vi "draw_rectangles.vi"(0 "Rectangle Array":dbl[][](array[numeric]), 1 "Robot Properties":T1, 2 "Sim Car.lvclass":refnum<class "Car.lvclass">) -> (7 "Map Picture":picture)   [LabVIEW 2015]
uses:
  Robot.ctl
  class/Car.lvclass
panel:
  out "x*y":dbl[](array[numeric])
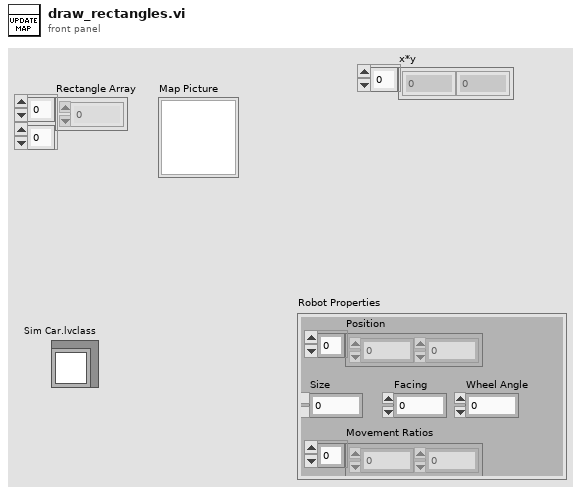
[diagram p1: front panel]
types:
  T1 = typedef "Robot.ctl" = cluster{"Position":dbl[], "Size":dbl, "Facing":dbl, "Movement Ratios":dbl[], "Wheel Angle":dbl}
  T2 = cluster{"Width":i16, "Style":enum32{"Solid", "Dash", "Dot", "DashDot", "DashDotDot"}}
  T3 = cluster{"Rectangle Array[0]":dbl, "Rectangle Array[1]":dbl, "Rectangle Array[2]":dbl, "Rectangle Array[3]":dbl}
  T4 = cluster{"Width":u16, "Style":enum32{"Solid", "Dash", "Dot", "DashDot", "DashDotDot"}}
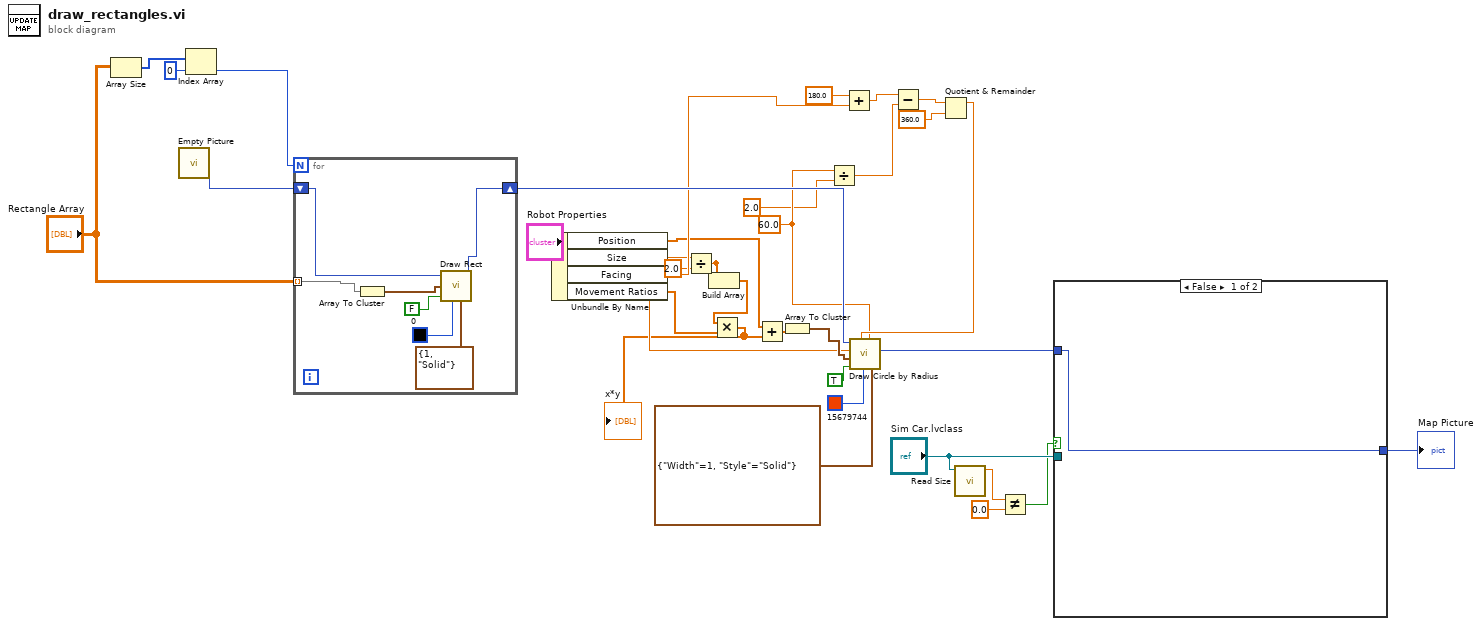
[diagram p0: block diagram]
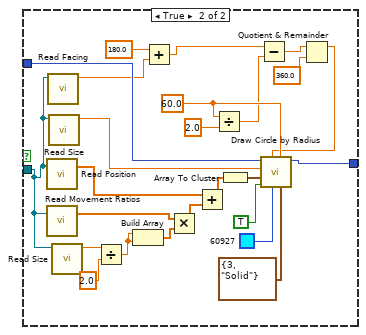
[diagram p2: hidden frame]
diagram:
  w19 = 60.0 ("arc size(360)")
  n1 = Array Size(array="Rectangle Array") -> (size(s)=w31:i32[])
  n2 = call "Empty Picture"() -> ("empty picture"=w34:picture)
  n3 = Index Array(array=w31, index=0) -> (element=w33:i32)
  n4 = for {
    N: w33 -> [_]
    tunnel: "Rectangle Array" -> [w41] mode=indexing
    shift-right: [w35] -> w29
    shift-left: w34 -> [w39]
    n5 = Array To Cluster(array=w41) -> (cluster=w40:T3)
    n6 = call <vilib>:"Draw Rect.vi"("picture"=w39, "rect"=w40, "fill?(F)"=FALSE, "color(black)"=u32 0, "pen"=T2 {"Width"=1, "Style"=enum."Solid"}) -> ("new picture"=w35:picture)  [unwired: 4 in]
  }
  n7 = Unbundle By Name("Robot Properties") -> ("Position"=w13:dbl[], "Size"=w11:dbl, "Facing"=w24:dbl, "Movement Ratios"=w7:dbl[])
  n8 = Divide(x=w11, y=2.0) -> (x/y=w10:dbl)
  n9 = Build Array(w10, w10) -> (w8:dbl[])
  n10 = Multiply(x=w8, y=w7) -> (x*y=w9:dbl[])
  "x*y" <- w9
  n11 = Add(x=w13, y=w9) -> (x+y=w14:dbl[])
  n12 = Array To Cluster(array=w14) -> (cluster=w15:cluster{"[0]":dbl, "[1]":dbl})
  n13 = Divide(x=w19, y=2.0) -> (x/y=w17:dbl)
  n14 = Add(x=180.0, y=w24) -> (x+y=w23:dbl)
  n15 = Subtract(x=w23, y=w17) -> (x-y=w22:dbl)
  n16 = Quotient & Remainder(x=w22, y=360.0) -> (x-y*floor(x/y)=w20:dbl)  [unwired: 1 out]
  n17 = call <vilib>:"Draw Circle by Radius.vi"("pen"=T2 {"Width"=1, "Style"=enum."Solid"}, "arc size(360)"=w19, "color(black)"=u32 15679744, "start angle(0)"=w20, "fill?(F)"=TRUE, "pixel center"=w15, "radius"=w11, "picture"=w29) -> ("new picture"=w6:picture)  [unwired: 3 in]
  n18 = call "Read Size.vi"("Car.lvclass"="Sim Car.lvclass") -> ("Size"=w3:dbl)  [unwired: 9 in, 1 out]
  n19 = Not Equal?(x=w3, y=0.0) -> (x != y?=w1:bool)
  n20 = case shown="False" w1 {
    tunnel: w6 -> [w42 w67]
    tunnel: [w42 w62] -> w5
    tunnel: "Sim Car.lvclass" -> [_ w43]
    frame False {
    }
    frame True {
      w50 = 60.0
      n21 = call "Read Position.vi"("Car.lvclass"=w43) -> ("Position"=w55:dbl[])  [unwired: 1 in, 1 out]
      n22 = call "Read Movement Ratios.vi"("Car.lvclass"=w43) -> ("Array"=w58:dbl[])  [unwired: 1 in, 1 out]
      n23 = call "Read Facing.vi"("Car.lvclass"=w43) -> ("Facing"=w52:dbl)  [unwired: 9 in, 1 out]
      n24 = call "Read Size.vi"("Car.lvclass"=w43) -> ("Size"=w66:dbl)  [unwired: 9 in, 1 out]
      n25 = call "Read Size.vi"("Car.lvclass"=w43) -> ("Size"=w60:dbl)  [unwired: 9 in, 1 out]
      n26 = Divide(x=w60, y=2.0) -> (x/y=w59:dbl)
      n27 = Build Array(w59, w59) -> (w57:dbl[])
      n28 = Add(x=180.0, y=w52) -> (x+y=w47:dbl)
      n29 = Multiply(x=w58, y=w57) -> (x*y=w56:dbl[])
      n30 = Add(x=w55, y=w56) -> (x+y=w54:dbl[])
      n31 = Divide(x=w50, y=2.0) -> (x/y=w48:dbl)
      n32 = Array To Cluster(array=w54) -> (cluster=w53:cluster{"[0]":dbl, "[1]":dbl})
      n33 = Subtract(x=w47, y=w48) -> (x-y=w46:dbl)
      n34 = Quotient & Remainder(x=w46, y=360.0) -> (x-y*floor(x/y)=w44:dbl)  [unwired: 1 out]
      n35 = call <vilib>:"Draw Circle by Radius.vi"("pen"=T4 {"Width"=3, "Style"=enum."Solid"}, "arc size(360)"=w50, "color(black)"=u32 60927, "start angle(0)"=w44, "fill?(F)"=TRUE, "pixel center"=w53, "radius"=w66, "picture"=w67) -> ("new picture"=w62:picture)  [unwired: 3 in]
    }
  }
  "Map Picture" <- w5
